vi "Autonomous shoot.vi"() -> (3 "Shot?":bool)   [LabVIEW 2015]
uses:
  Robot Values.vi
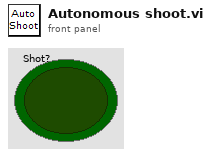
[diagram p1: front panel]
types:
  T1 = typedef "Robot Values.ctl" = cluster{"Drive Motors":cluster{"Left Motor Value":dbl, "Right Motor Value":dbl, "Left Motor Encoder":dbl, "Right Motor Encoder":dbl, "High/Low Gear":bool}, "Sensors":cluster{"Gyro Angle":dbl, "Photoeye":bool, "Ultrasonic Range":dbl, "Shooter Speed Encoder":dbl, "Accelerometer Value":dbl, "Flashlight":bool, "Target Distance":dbl, "Target X Value":dbl, "Reset Gyro?":bool}, "Arms":cluster{"Desired Arm Position":dbl, "Left Arm Encoder":dbl, "Right Arm Encoder":dbl, "Left Arm Lower Limit":bool, "Right Arm Lower Limit":bool, "Initialize Arm Position?":bool}, "Acquisition and Scoring":cluster{"Acquiring?":bool, "Current Speed":dbl, "Setpoint Speed":dbl, "Prep Wheels":bool, "Shoot":bool, "Low Eject":bool, "Reverse Shooter Wheel":bool}, "Hanging":cluster{"Pivot Arms":dbl, "PTO":bool, "Left Pivot Encoder":dbl, "Right Pivot Encoder":dbl, "Hanging Pin":bool}}
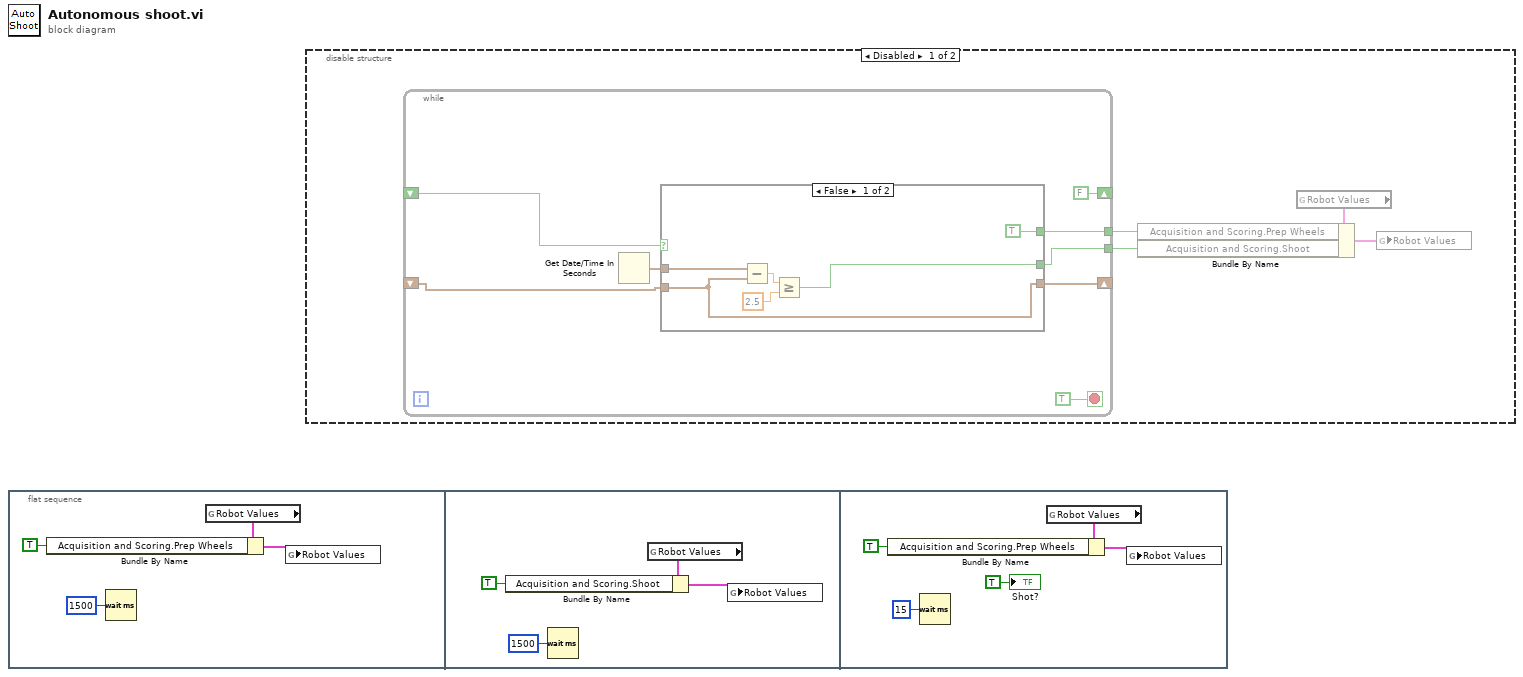
[diagram p0: block diagram]
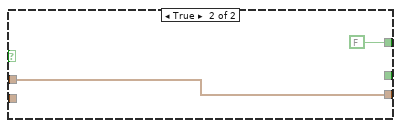
[diagram p2: hidden frame]
diagram:
  n1 = flat-sequence {
    frame #0 {
      n2 = Wait (ms)(milliseconds to wait=u32 1500) -> ()  [unwired: 1 out]
      n3 = global read "Robot Values.vi" "Robot Values"() -> (w3:T1)
      n4 = Bundle By Name(cluster=w3, "Acquisition and Scoring.Prep Wheels"=TRUE) -> (w4:T1)
      n5 = global write "Robot Values.vi" "Robot Values"(w4) -> ()
    }
    frame #1 {
      n6 = Wait (ms)(milliseconds to wait=u32 1500) -> ()  [unwired: 1 out]
      n7 = global read "Robot Values.vi" "Robot Values"() -> (w7:T1)
      n8 = Bundle By Name(cluster=w7, "Acquisition and Scoring.Shoot"=TRUE) -> (w8:T1)
      n9 = global write "Robot Values.vi" "Robot Values"(w8) -> ()
    }
    frame #2 {
      n10 = Wait (ms)(milliseconds to wait=u32 15) -> ()  [unwired: 1 out]
      n11 = global read "Robot Values.vi" "Robot Values"() -> (w11:T1)
      n12 = Bundle By Name(cluster=w11, "Acquisition and Scoring.Prep Wheels"=TRUE) -> (w12:T1)
      n13 = global write "Robot Values.vi" "Robot Values"(w12) -> ()
      "Shot?" <- TRUE ("Shot?")
    }
  }
  n14 = disable-structure shown="Disabled" {
    frame Disabled {
      n15 = while {
        shift-right: [w24] -> _
        shift-left: _ -> [w23]
        tunnel: [w21] -> w14
        tunnel: [w20] -> w15
        shift-right: [FALSE ("First Call?")] -> _
        shift-left: _ -> [w19]
        stop <- TRUE stop-if-true
        n16 = Get Date/Time In Seconds() -> (seconds since 1Jan1904=w22:timestamp)
        n17 = case shown="False" w19 {
          tunnel: w22 -> [w31 w33]
          tunnel: [w27 w33] -> w24
          tunnel: w23 -> [w27 _]
          tunnel: [w28 _] -> w21
          tunnel: [TRUE FALSE] -> w20
          frame False {
            n18 = Subtract(x=w31, y=w27) -> (x-y=w30:dbl)
            n19 = Greater Or Equal?(x=w30, y=2.5) -> (x >= y?=w28:bool)
          }
          frame True {
          }
        }
      }
      n20 = global read "Robot Values.vi" "Robot Values"() -> (w16:T1)
      n21 = Bundle By Name(cluster=w16, "Acquisition and Scoring.Prep Wheels"=w15, "Acquisition and Scoring.Shoot"=w14) -> (w17:T1)
      n22 = global write "Robot Values.vi" "Robot Values"(w17) -> ()
    }
    frame Enabled {
    }
  }
